vi "ProdaNG.Products.Get.vi"(5 "Time To":string, 7 "Time From":string, 8 "error in (no error)":errorcluster, 9 "proccessStepId (0: all)":i32, 10 "wabcoPartId":i32, 11 "dbHandleIn":i32) -> (0 "error out":errorcluster, 1 "Serials":string[](array[string]), 2 "Products":T1[](array[typedef]), 3 "dbHandle":i32)   [LabVIEW 2016]
doc: "This function returns a product structure for a product, which is identified by a part and a serial number.\nImportant information: The field 'individual' was taken over from the field 'allgemein' of the legacy data directly. Because of this most products have the value 0 further on and only a few the value 1. \nParameter:\nhandle is an Integer, which is returned by the function Login() at the creation of a new connection.\nwabcoPartId is the Id of the part.\nserialNumber is the serial number of the product for the part above.\nproduct is a pointer on a product structure, which is filled if the returncode is 0. The structure must be defined in the calling program.\n\nReturncodes:\n0 No error\n< 0 ORACLE Error code\n6 (ERROR_INVALID_HANDLE) in case of an invalid handle\n1403 Record does not exist"
uses:
  Controls/ProdaNG.Product.ctl
  Controls/ProdaNG.ProductSize.ctl
  <vilib>/Utility/importsl/GetValueByPointer/datatype.ctl
  <vilib>/Utility/importsl/GetValueByPointer/GetValueByPointer.xnode
  prodllNG.dll
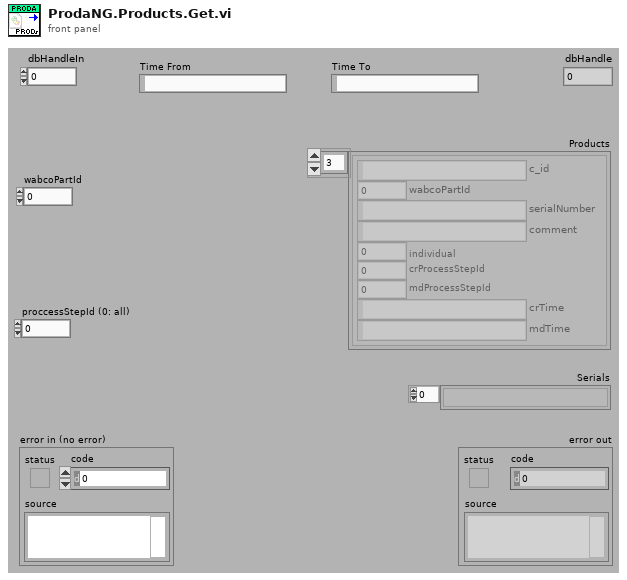
[diagram p1: front panel]
types:
  T1 = typedef "ProdaNG.Product.ctl" = cluster{"c_id":string, "wabcoPartId":i32, "serialNumber":string, "comment":string, "individual":i32, "crProcessStepId":i32, "mdProcessStepId":i32, "crTime":string, "mdTime":string}
  T2 = typedef "ProdaNG.ProductSize.ctl" = cluster{"c_id":i32, "wabcoPartId":i32, "serialNumber":i32, "comment":i32, "individual":i32, "crProcessStepId":i32, "mdProcessStepId":i32, "crTime":i32, "mdTime":i32}
  T3 = cluster{"LV string":string, "LV string":string, "Product":T1}
  T4 = cluster{"LV string":string, "LV string":string, "Product":T1}[]
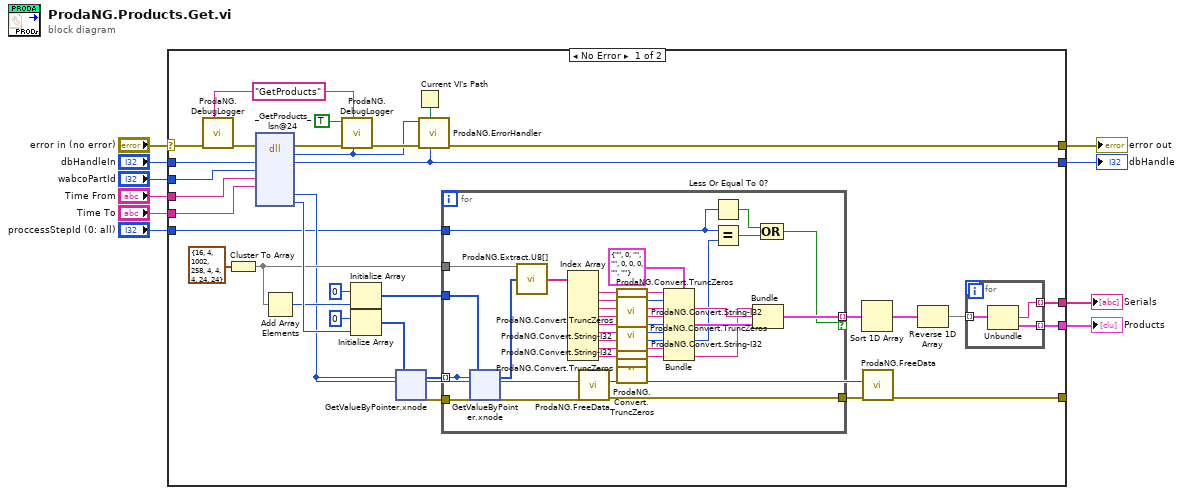
[diagram p0: block diagram]
diagram:
  n1 = case shown="No Error" "error in (no error)" {
    selector: "error in (no error)" -> [w38 w111]
    tunnel: [w43 w111] -> w9
    tunnel: "dbHandleIn" -> [w40 w110]
    tunnel: [w41 w110] -> w7
    tunnel: "wabcoPartId" -> [w25 _]
    tunnel: [w17 _] -> w5
    tunnel: [w20 _] -> _
    tunnel: "Time From" -> [w15 _]
    tunnel: "Time To" -> [w14 _]
    tunnel: [w13 _] -> w2
    tunnel: "proccessStepId (0: all)" -> [w11 _]
    frame No Error {
      w34 = "GetProducts" ("cmd")
      n2 = call "ProdaNG.DebugLogger.vi"("cmd"=w34, "error in (no error)"=w38) -> ("error out"=w37:errorcluster)  [unwired: 9 in]
      n3 = Cluster To Array(cluster=T2 {"c_id"=16, "wabcoPartId"=4, "serialNumber"=1002, "comment"=258, "individual"=4, "crProcessStepId"=4, "mdProcessStepId"=4, "crTime"=24, "mdTime"=24} ("ProductSize")) -> (array=w23:i32[])
      n4 = dll-call lib="D:/Maszup/WABCO/SVN/LineTraceSystem/SOFTWARE/sources/Database/ProdaNG/prodllNG.dll" fn="_GetProducts_lsn@24" ("ProDLL wrapper.dll:ProDLL_wrapper_GetWabcoParts_GetData")(error in=w37, "dbHandle"=w40, "wabcoPartId"=w25, "crTime1"=w15, "crTime2"=w14) -> (error out=w36:errorcluster, "return type"=w33:i32, "dbHandle"=w41:i32, "products"=w19:u32, "countPtr"=w28:i32)  [unwired: 7 in, 1 out]
      n5 = Add Array Elements(numeric array=w23) -> (sum=w24:i32)
      n6 = call "ProdaNG.DebugLogger.vi"("return type"=w33, "cmd"=w34, "error in (no error)"=w36, "done? (F)"=TRUE) -> ("error out"=w35:errorcluster)  [unwired: 7 in]
      n7 = Initialize Array(u8 0 ("element"), w24) -> (w26:u8[])
      n8 = Initialize Array(u32 0 ("element"), w28) -> (w32:u32[])
      n9 = xnode "GetValueByPointer.xnode"("Pointer"=w19, "InputType"=w32) -> ("Output"=w29:u32[], "ErrorOut"=w30:errorcluster)  [unwired: 2 in]
      n10 = Current VI's Path() -> (path=w42:path)
      n11 = call "ProdaNG.ErrorHandler.vi"("dbHandleIn"=w41, "Path"=w42, "error in"=w35, "output_parameter"=w33) -> ("error out"=w43:errorcluster)  [unwired: 7 in]
      n12 = for {
        tunnel: w30 -> [w79]
        tunnel: w29 -> [w74] mode=indexing
        tunnel: w26 -> [w78]
        tunnel: w23 -> [w76]
        tunnel: [w72] -> w22 mode=indexing if=w48
        tunnel: [w73] -> w21
        tunnel: w11 -> [w51]
        n13 = xnode "GetValueByPointer.xnode"("Pointer"=w74, "InputType"=w78, "ErrorIn"=w79) -> ("Output"=w77:u8[], "ErrorOut"=w75:errorcluster)  [unwired: 1 in]
        n14 = call "ProdaNG.Extract.U8[].vi"("unsigned byte array"=w77, "Sizes"=w76) -> ("Elements"=w56:string[])
        n15 = Index Array(array=w56) -> (element #1=w58:string, element #2=w69:string, element #3=w63:string, element #4=w62:string, element #5=w68:string, element #6=w66:string, element #7=w64:string, element #8=w60:string, element #9=w59:string)  [unwired: 9 in]
        n16 = call "ProdaNG.FreeData.vi"("error in (no error)"=w75, "Pointers"=w74) -> ("error out"=w73:errorcluster)  [unwired: 9 in]
        n17 = call "ProdaNG.Convert.TruncZeros.vi"("string with \\0s"=w58) -> ("LV string"=w57:string)  [unwired: 10 in]
        n18 = call "ProdaNG.Convert.String-I32.vi"("unsigned byte string"=w69) -> ("32bit integer"=w70:i32)  [unwired: 10 in]
        n19 = call "ProdaNG.Convert.TruncZeros.vi"("string with \\0s"=w63) -> ("LV string"=w53:string)  [unwired: 10 in]
        n20 = call "ProdaNG.Convert.TruncZeros.vi"("string with \\0s"=w62) -> ("LV string"=w61:string)  [unwired: 10 in]
        n21 = call "ProdaNG.Convert.String-I32.vi"("unsigned byte string"=w68) -> ("32bit integer"=w67:i32)  [unwired: 10 in]
        n22 = call "ProdaNG.Convert.String-I32.vi"("unsigned byte string"=w66) -> ("32bit integer"=w65:i32)  [unwired: 10 in]
        n23 = call "ProdaNG.Convert.String-I32.vi"("unsigned byte string"=w64) -> ("32bit integer"=w52:i32)  [unwired: 10 in]
        n24 = call "ProdaNG.Convert.TruncZeros.vi"("string with \\0s"=w60) -> ("LV string"=w54:string)  [unwired: 10 in]
        n25 = call "ProdaNG.Convert.TruncZeros.vi"("string with \\0s"=w59) -> ("LV string"=w47:string)  [unwired: 10 in]
        n26 = Bundle(cluster=T1 {"c_id"="", "wabcoPartId"=0, "serialNumber"="", "comment"="", "individual"=0, "crProcessStepId"=0, "mdProcessStepId"=0, "crTime"="", "mdTime"=""} ("Product"), "c_id"=w57, "wabcoPartId"=w70, "serialNumber"=w53, "comment"=w61, "individual"=w67, "crProcessStepId"=w65, "mdProcessStepId"=w52, "crTime"=w54, "mdTime"=w47) -> (w55:T1)
        n27 = Less Or Equal To 0?(x=w51) -> (x <= 0?=w49:bool)
        n28 = Equal?(x=w51, y=w52) -> (x = y?=w50:bool)
        n29 = Bundle("LV string"=w47, "LV string"=w53, "Product"=w55) -> (w72:T3)  [unwired: 1 in]
        n30 = Compound Arithmetic op=OR(w49, w50) -> (w48:bool)
      }
      n31 = Sort 1D Array(array=w22) -> (sorted array=w18:T4)
      n32 = call "ProdaNG.FreeData.vi"("error in (no error)"=w21, "Pointers"=w19) -> ("error out"=w20:errorcluster)  [unwired: 9 in]
      n33 = Reverse 1D Array(array=w18) -> (reversed array=w12:T4)
      n34 = for {
        tunnel: w12 -> [w46] mode=indexing
        tunnel: [w45] -> w17 mode=indexing
        tunnel: [w44] -> w13 mode=indexing
        n35 = Unbundle(w46) -> ("LV string"=w44:string, "Product"=w45:T1)  [unwired: 1 out]
      }
    }
    frame Error {
    }
  }
  "error out" <- w9
  "dbHandle" <- w7
  "Products" <- w5
  "Serials" <- w2
